vi "test_ubx-format.vi"() -> ()   [LabVIEW 2019]
uses:
  Ctrl/ubx-packet.ctl
panel:
  out "crc final 2":u32 format="%x"
  in  "인덱스":i32
  out "crc val":bool
  out "crc final":u8 format="%x"
  out "crc cal":u8 format="%x"
  out "ubx arr":T1[](array[typedef])
  out "crc":u8[](array[numeric])=[211, 0, 126, 254, 128, 0, 1, 0, 0, 22, 215, 14, 230, 64, 7, 28, 198, 123, 137, 228, 184, 99, 200, 223, 145, 240, 78, 205, 125, 255, 255, 68, 0, 0, 155, 255, 254, 227, 255, 255, 255, 98, 0, 0, 1, 64, 0, 0, 2, 63, 67, 72, 127, 255, 255, 148, 33, 93, 31, 255, 255, 238, 71, 73, 64, 0, 0, 7, 205, 79, 216, 0, 0, 1, 58, 198, 194, 0, 0, 0, 188, 232, 73, 0, 0, 0, 9, 49, 173, 63, 255, 255, 250, 6, 47, 128, 0, 0, 9, 197, 77, 0, 0, 0, 50, 250, 77, 255, 255, 255, 242, 14, 192, 0, 0, 1, 91, 98, 128, 0, 0, 249, 224, 0, 0, 34] format="%02x"
  out "next str":string
  out "숫자":u32=126 format="%x"
  out "불리언 배열":bool[](array[boolean])
  out "rtcm data":u8[](array[numeric])=[211, 0, 126, 254, 128, 0, 1, 0, 0, 22, 215, 14, 230, 64, 7, 28, 198, 123, 137, 228, 184, 99, 200, 223, 145, 240, 78, 205, 125, 255, 255, 68, 0, 0, 155, 255, 254, 227, 255, 255, 255, 98, 0, 0, 1, 64, 0, 0, 2, 63, 67, 72, 127, 255, 255, 148, 33, 93, 31, 255, 255, 238, 71, 73, 64, 0, 0, 7, 205, 79, 216, 0, 0, 1, 58, 198, 194, 0, 0, 0, 188, 232, 73, 0, 0, 0, 9, 49, 173, 63, 255, 255, 250, 6, 47, 128, 0, 0, 9, 197, 77, 0, 0, 0, 50, 250, 77, 255, 255, 255, 242, 14, 192, 0, 0, 1, 91, 98, 128, 0, 0, 249, 224, 0, 0, 34, 216, 0, 0, 181, 18, 161, 36] format="%02x"
  in  "nmea":string="Ø\u0000\u0000µ\u0012¡$GNGGA,073011.40,3723.65976,N,12656.93446,E,1,12,0.53,70.3,M,18.5,M,,*7B\r\n"
  in  "RTCM3":string="Ó\u0000~þ€\u0000\u0001\u0000\u0000\u0016×\u000eæ@\u0007\u001cÆ{‰ä¸cÈß‘ðNÍ}ÿÿD\u0000\u0000›ÿþãÿÿÿb\u0000\u0000\u0001@\u0000\u0000\u0002?CHÿÿ”!]\u001fÿÿîGI@\u0000\u0000\u0007ÍOØ\u0000\u0000\u0001:ÆÂ\u0000\u0000\u0000¼èI\u0000\u0000\u0000\t1­?ÿÿú\u0006/€\u0000\u0000\tÅM\u0000\u0000\u00002úMÿÿÿò\u000eÀ\u0000\u0000\u0001[b€\u0000\u0000ùà\u0000\u0000\"Ø\u0000\u0000µ\u0012¡$"
  in  "read_buffer":string
  # "B562 0107 5C00 983B 5C1B E507 0101 071E 0B37 0300 0000 C5FF D917 0301 EA1C B5DD AA4B FDEB 4916 D75A 0100 A312 0100 5103 0000 0F05 0000 EDFF FFFF 0300 0000 FFFF FFFF 1300 0000 A912 6A00 BB00 0000 8EBB 9300 6200 0000 BA65 432C 0000 0000 0000 0000 8A6A"
  # "B562 013B 2800 0000 0000 983B 5C1B 0000 0000 0000 0000 0000 0000 0000 0000 0000 0000 0000 0000 0000 0000 0000 0000 AEC9"
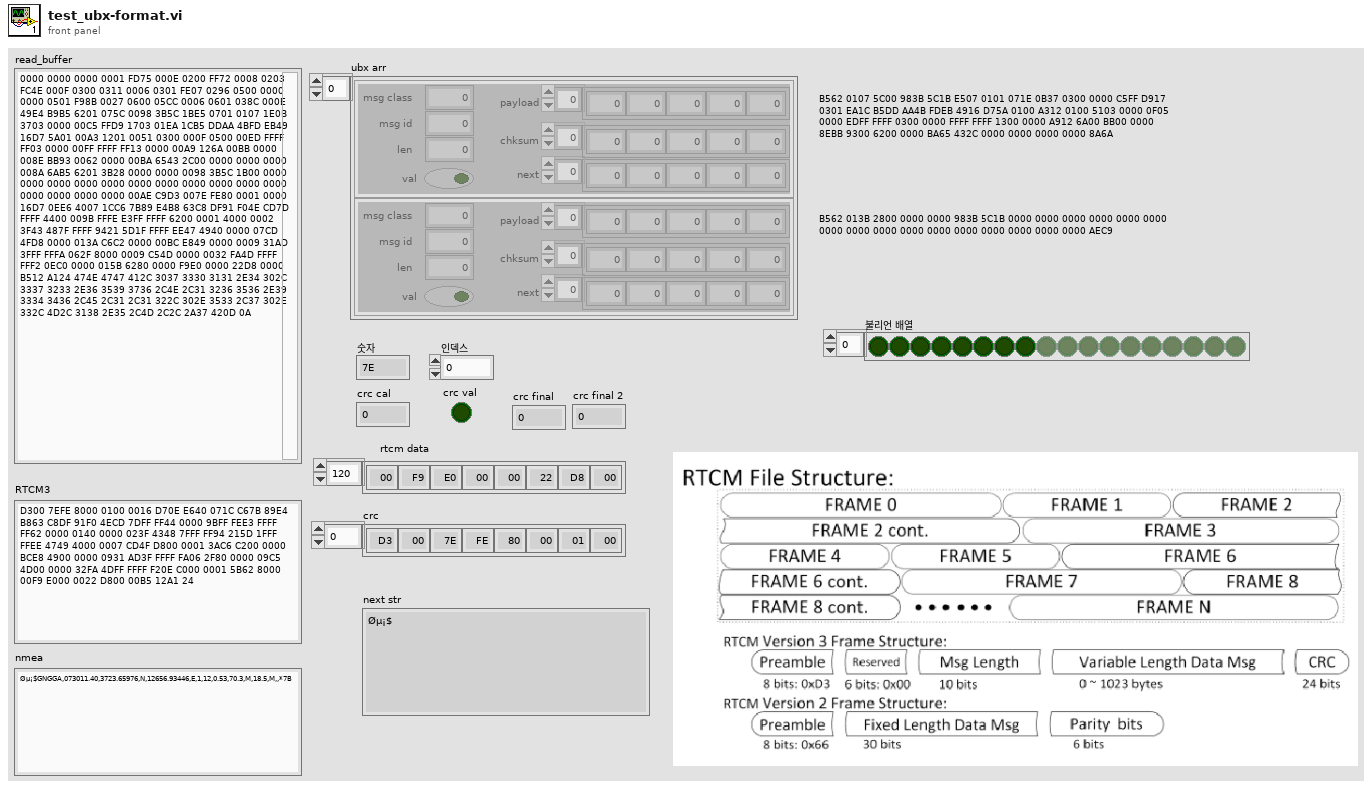
[diagram p1: front panel]
types:
  T1 = typedef "ubx-packet.ctl" = cluster{"msg class":u8, "msg id":u8, "len":u8, "payload":u8[], "chksum":u8[], "next ":u8[], "val":bool}
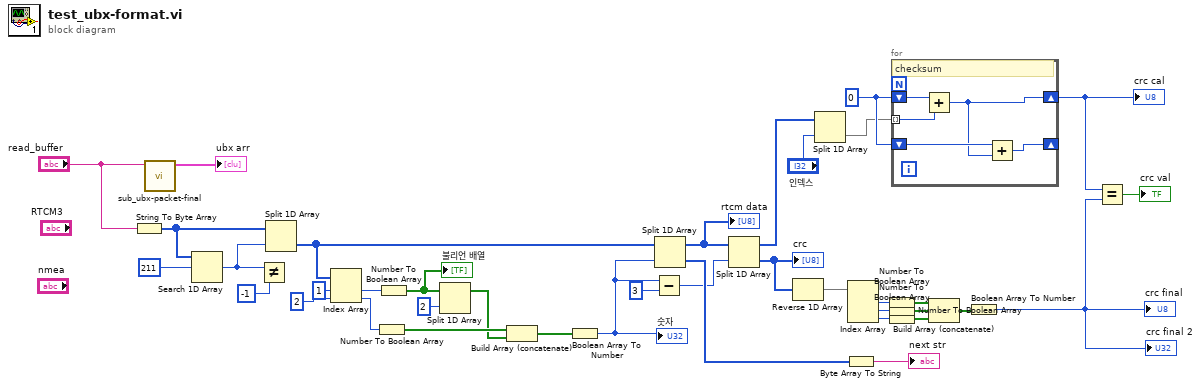
[diagram p0: block diagram]
diagram:
  w17 = u8 0 ("y")
  n1 = String To Byte Array(string="read_buffer") -> (unsigned byte array=w35:u8[])
  n2 = call "sub_ubx-packet-final.vi"("read_buffer"="read_buffer") -> ("ubx pk arr"=→"ubx arr":T1[])  [unwired: 10 in]
  n3 = Search 1D Array(1D array=w35, element=u8 211 ("rtcm preamble")) -> (index of element=w36:i32)  [unwired: 1 in]
  n4 = Not Equal?(x=w36, y=-1) -> ()  [unwired: 1 out]
  n5 = Split 1D Array(array=w35, index=w36) -> (second subarray=w25:u8[])  [unwired: 1 out]
  n6 = Index Array(array=w25, index #1=1 ("인덱스"), index #2=2 ("인덱스")) -> (element #1=w32:u8, element #2=w31:u8)
  n7 = Number To Boolean Array(number=w31) -> (Boolean array=w28:bool[])
  n8 = Number To Boolean Array(number=w32) -> (Boolean array=w30:bool[])
  "불리언 배열" <- w30
  n9 = Split 1D Array(array=w30, index=2 ("인덱스")) -> (first subarray=w27:bool[])  [unwired: 1 out]
  n10 = Build Array (concatenate)(w28, w27) -> (w26:bool[])
  n11 = Boolean Array To Number(Boolean array=w26) -> (number=w21:u32)
  "숫자" <- w21
  n12 = Subtract(x=w21, y=u32 3) -> (x-y=w22:u32)
  n13 = Split 1D Array(array=w25, index=w21) -> (first subarray=w16:u8[], second subarray=w23:u8[])
  "rtcm data" <- w16
  n14 = Split 1D Array(array=w16, index=w22) -> (first subarray=w4:u8[], second subarray=w15:u8[])
  "crc" <- w15
  n15 = Reverse 1D Array(array=w15) -> (reversed array=w11:u8[])
  n16 = Split 1D Array(array=w4, index="인덱스") -> (second subarray=w2:u8[])  [unwired: 1 out]
  n17 = Byte Array To String(unsigned byte array=w23) -> (string=→"next str":string)
  n18 = Index Array(array=w11) -> (element #1=w14:u8, element #2=w13:u8, element #3=w12:u8)  [unwired: 3 in]
  n19 = Number To Boolean Array(number=w14) -> (Boolean array=w8:bool[])
  n20 = Number To Boolean Array(number=w13) -> (Boolean array=w9:bool[])
  n21 = Number To Boolean Array(number=w12) -> (Boolean array=w10:bool[])
  n22 = for {
    tunnel: w2 -> [w43] mode=indexing
    shift-right: [w40] -> w6
    shift-left: w17 -> [w42]
    shift-right: [w39] -> _
    shift-left: w17 -> [w41]
    # "checksum"
    n23 = Add(x=w42, y=w43) -> (x+y=w40:u8)
    n24 = Add(x=w41, y=w40) -> (x+y=w39:u8)
  }
  "crc cal" <- w6
  n25 = Build Array (concatenate)(w8, w9, w10) -> (w7:bool[])
  n26 = Boolean Array To Number(Boolean array=w7) -> (number=w1:u32)
  "crc final" <- w1
  "crc final 2" <- w1
  n27 = Equal?(x=w6, y=w1) -> (x = y?=→"crc val":bool)
